vi "comms_Serial_Read_TXT.vi"(8 "error in":errorcluster, 11 "VISA resource in":refnum<visa-resource-name>) -> (0 "error out":errorcluster, 1 "Read Count":i32, 2 "Data Out":string, 3 "VISA resource Out":refnum<visa-resource-name>)   [LabVIEW 2016]
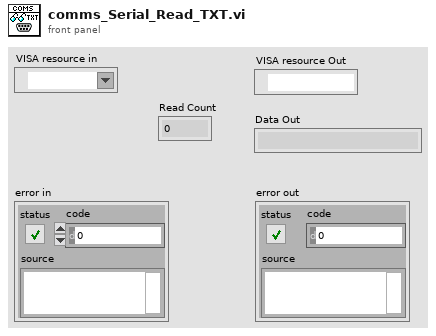
[diagram p1: front panel]
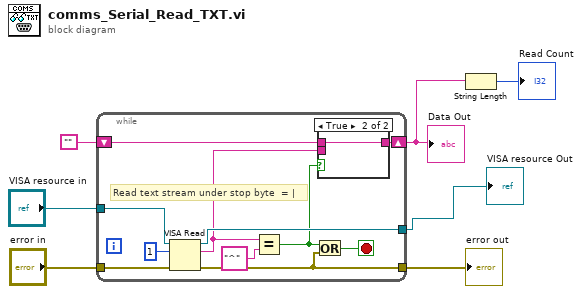
[diagram p0: block diagram]
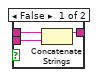
[diagram p2: hidden frame]
diagram:
  n1 = while {
    tunnel: "VISA resource in" -> [w17]
    tunnel: [w15] -> w5
    tunnel: [w14] -> w4
    tunnel: "error in" -> [w13]
    shift-right: [w9] -> w3
    shift-left: "" -> [w11]
    stop <- w16 stop-if-true
    # "Read text stream under stop byte  = |"
    n2 = VISA Read(VISA resource name=w17, byte count=u32 1, error in (no error)=w13) -> (VISA resource name out=w15:refnum<visa-resource-name>, read buffer=w10:string, error out=w14:errorcluster)  [unwired: 1 out]
    n3 = Equal?(x=w10, y="^") -> (x = y?=w8:bool)
    n4 = Or(x=w8, y=w14) -> (x .or. y?=w16:bool)
    n5 = case shown="True" w8 {
      tunnel: w11 -> [w21 w22]
      tunnel: w10 -> [w20 _]
      tunnel: [w19 w22] -> w9
      frame False {
        n6 = Concatenate Strings(w21, w20) -> (w19:string)
      }
      frame True {
      }
    }
  }
  "VISA resource Out" <- w5
  "error out" <- w4
  "Data Out" <- w3
  n7 = String Length(string=w3) -> (length=→"Read Count":i32)
